vi "PlotSingleOHcube_ILThack.vi"() -> ()   [LabVIEW 2014]
uses:
  TypeDefs/RectHatch.ctl
  TypeDefs/PowerSpeed.ctl
panel:
  in  "OHpows":dbl[](array[numeric])=[50.0, 75.0, 100.0, 125.0, 250.0]
  in  "EndLayer":u32=170
  in  "Display":T1={"Mode"=enum."Inherit Value", "PointSize"=1.0, "LineWidth"=1.0}
  in  "HighPower":dbl=500.0
  in  "StartLayer":u32=170
  in  "HatchPow":T2={"Power"=300.0, "Mark Speed"=400.0, "Jump Speed"=1000.0}
  in  "RectHatch":T3={"Width"=10.0, "Height"=10.0, "Angle"=45.0, "OffX"=0.1, "OffY"=0.1, "Spacing"=0.1} {"Spacing" format="%#_13g"; "OffY" format="%#_13g"; "OffX" format="%#_13g"; "Height" format="%#_13g"; "Width" format="%#_13g"}
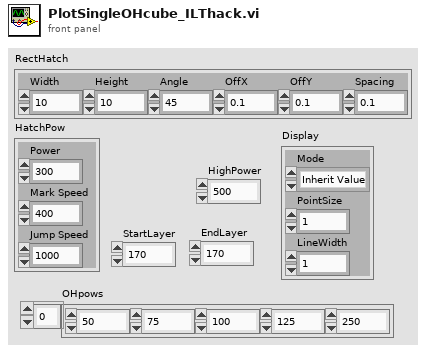
[diagram p1: front panel]
types:
  T1 = cluster{"Mode":enum16{"Inherit Value", "Points", "Wireframe", "Polygons"}, "PointSize":sgl, "LineWidth":sgl}
  T2 = typedef "PowerSpeed.ctl" = cluster{"Power":dbl, "Mark Speed":dbl, "Jump Speed":dbl}
  T3 = typedef "RectHatch.ctl" = cluster{"Width":dbl, "Height":dbl, "Angle":sgl, "OffX":dbl, "OffY":dbl, "Spacing":dbl}
  T4 = cluster{"Start":cluster{"X":dbl, "Y":dbl}, "End":cluster{"X":dbl, "Y":dbl}}[]
  T5 = typedef "PathSupreme.ctl" = cluster{"VelocityProfiles":T6[], "Path":T7}
  T6 = typedef "VelocityProfile.ctl" = cluster{"ID":u32, "Velocity":dbl, "Mode":string, "tV1":u32, "tV2":u32, "tL1":u32, "tL2":u32}
  T7 = typedef "PathCut.ctl" = cluster{"Type":string, "Tag":string, "Segments":T8[]}
  T8 = typedef "Segment.ctl" = cluster{"SegmentID":u16, "Power":sgl, "idxVelocityProfile":u16, "End":cluster{"X":sgl, "Y":sgl}}
  T9 = typedef "Point3D.ctl" = cluster{"X":sgl, "Y":sgl, "Z":sgl}
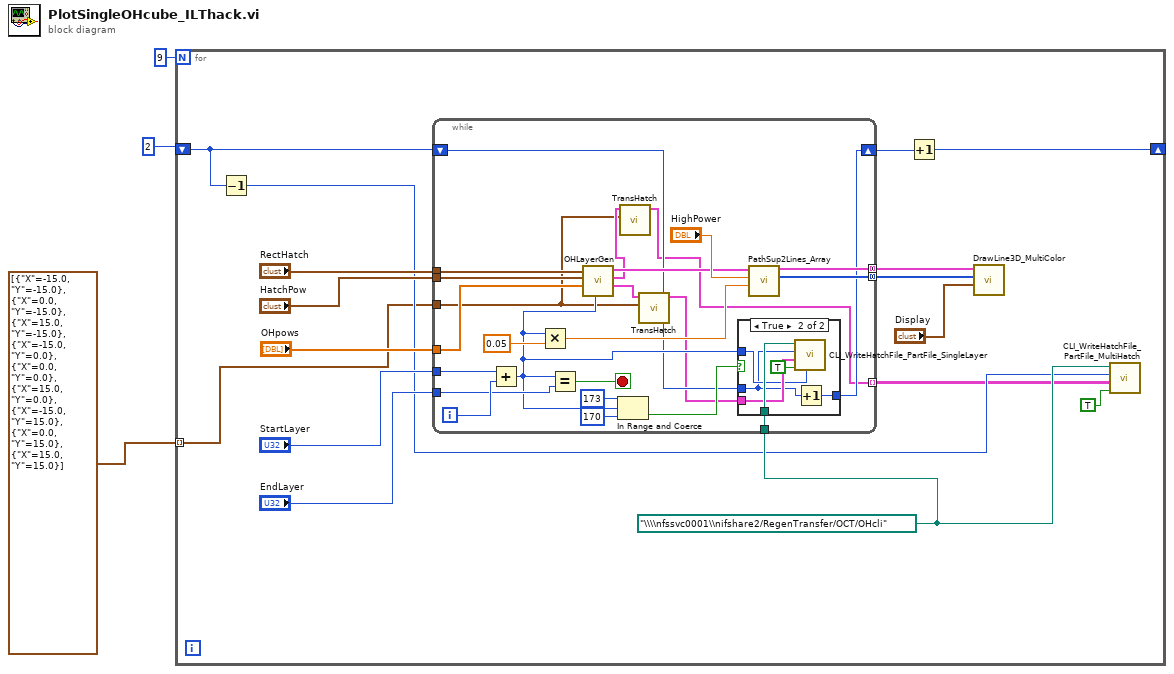
[diagram p0: block diagram]
diagram:
  n1 = for {
    N: 9 -> [_]
    shift-right: [w4] -> _
    shift-left: 2 -> [w9]
    tunnel: cluster{"X":dbl, "Y":dbl}[] [{"X"=-15.0, "Y"=-15.0}, {"X"=0.0, "Y"=-15.0}, {"X"=15.0, "Y"=-15.0}, {"X"=-15.0, "Y"=0.0}, {"X"=0.0, "Y"=0.0}, {"X"=15.0, "Y"=0.0}, {"X"=-15.0, "Y"=15.0}, {"X"=0.0, "Y"=15.0}, {"X"=15.0, "Y"=15.0}] -> [w7] mode=indexing
    w10 = path "\\\\nfssvc0001\\nifshare2/RegenTransfer/OCT/OHcli" ("Path")
    n2 = Decrement(x=w9) -> (x-1=w8:i32)
    n3 = while {
      tunnel: [w44] -> w19 mode=concatenating
      tunnel: [w43] -> w18 mode=concatenating
      tunnel: "RectHatch" -> [w42]
      tunnel: "HatchPow" -> [w41]
      tunnel: "StartLayer" -> [w37]
      tunnel: "EndLayer" -> [w35]
      tunnel: "OHpows" -> [w32]
      tunnel: [w20] -> w6 mode=indexing
      tunnel: w10 -> [w29]
      shift-right: [w25] -> w5
      shift-left: w9 -> [w26]
      tunnel: w7 -> [w21]
      i -> [w36]
      stop <- w38 stop-if-true
      n4 = Add(x=w37, y=w36) -> (x+y=w28:u32)
      n5 = Multiply(x=w28, y=0.05) -> (x*y=w34:dbl)
      n6 = Equal?(x=w28, y=w35) -> (x = y?=w38:bool)
      n7 = call "OHLayerGen.vi"("Layer"=w28, "OHpows"=w32, "HatchPow"=w41, "RectHatch"=w42) -> ("Hatches2"=w24:T4, "Hatches"=w22:T4, "PathSups"=w33:T5[])  [unwired: 5 in]
      n8 = In Range and Coerce(upper limit=u32 173, x=w28, lower limit=u32 170) -> (In Range?=w27:bool)  [unwired: 1 out]
      n9 = call "TransHatch.vi"("Offset"=w21, "HatchesIn"=w22) -> ("HatchesOut"=w20:T4)  [unwired: 9 in]
      n10 = call "TransHatch.vi"("Offset"=w21, "HatchesIn"=w24) -> ("HatchesOut"=w23:T4)  [unwired: 9 in]
      n11 = case shown="True" w27 {
        tunnel: w29 -> [_ w51]
        tunnel: w23 -> [_ w50]
        tunnel: w28 -> [_ w48]
        tunnel: w26 -> [w45 w46]
        tunnel: [w45 w47] -> w25
        frame False {
        }
        frame True {
          n12 = call "CLI_WriteHatchFile_PartFile_SingleLayer.vi"("Layer"=w48, "Write?"=TRUE, "Hatches"=w50, "PartNum"=w46, "Path"=w51) -> ()  [unwired: 6 in, 1 out]
          n13 = Increment(x=w46) -> (x+1=w47:i32)
        }
      }
      n14 = call "PathSup2Lines_Array.vi"("Z"=w34, "HighPower"="HighPower", "PathSupIn"=w33) -> ("Colors"=w43:u32[], "Lines"=w44:cluster{"P0":T9, "P1":T9}[])  [unwired: 7 in]
    }
    n15 = Increment(x=w5) -> (x+1=w4:i32)
    n16 = call "DrawLine3D_MultiColor.vi"("Display"="Display", "Colors"=w18, "Lines"=w19) -> ()  [unwired: 9 in]
    n17 = call "CLI_WriteHatchFile_PartFile_MultiHatch.vi"("Write?"=TRUE, "Hatches"=w6, "PartNum"=w8, "Path"=w10) -> ()  [unwired: 7 in, 1 out]
  }
